vi "TestPython.vi"(8 "error in (no error)":errorcluster, 11 "Py Session":refnum<k35>) -> (0 "error out":errorcluster, 3 "Py Session out":refnum<k35>)   [LabVIEW 2022 SP3, in "DLP2.lvclass"]
uses:
  DLP2.lvclass
  DLP2.lvclass/DLP2.ctl
panel:
  out "return value":i32
  out "Cluster":cluster{"Error":bool, "Status":string}
  # "python PPP_app_CLI.py -t C30L -p DL_1 -ph 1 -m C30L -w 0.0898 -d 1.00 -o 1.15 -x 5 -n 735957 -f DB -l None -z True -c compensation_zone_list2.csv -b WBG_images\\DL_1_C30L.bmp -r True -s cwd\\Dithered_images -g cwd\\Saved_GS_images -ro True -dr \"SQL Server\" -se tt-local.digilens.com -db ToolTrack -u tooltrack-user -pa DigiLens_rEAd_passwrd"
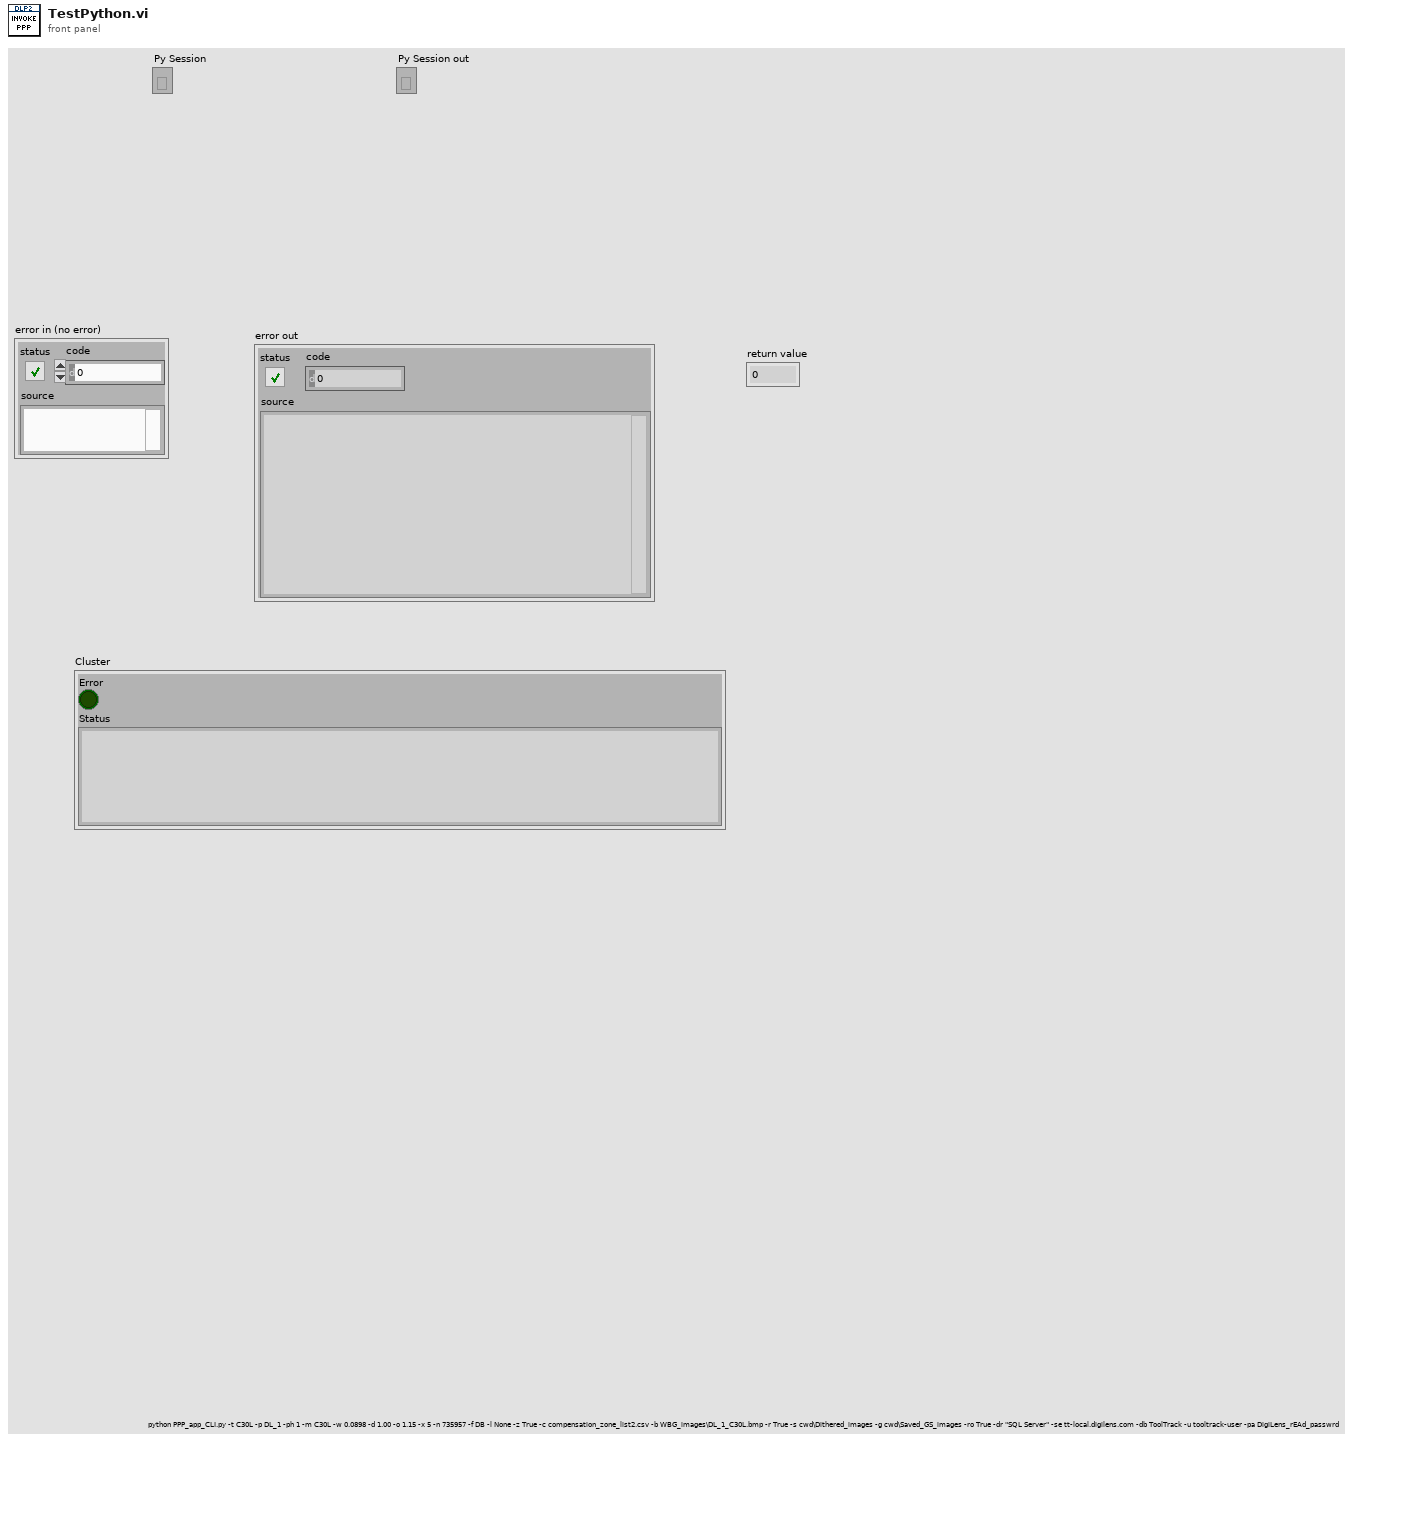
[diagram p1: front panel]
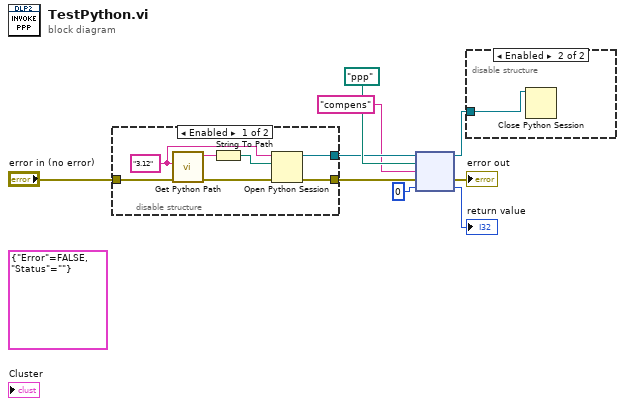
[diagram p0: block diagram]
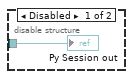
[diagram p2: hidden frame]
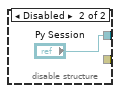
[diagram p3: hidden frame]
diagram:
  (unwired) cluster{"Error":bool, "Status":string} {"Error"=FALSE, "Status"=""}
  n1 = disable-structure shown="Enabled" {
    disable-tunnel: [w13 "Py Session"] -> w6
    disable-tunnel: [w12 _] -> w5
    disable-tunnel: "error in (no error)" -> [w10 _]
    frame Enabled {
      w14 = "3.12" ("Python Rev Key")
      n2 = call "Get Python Path.vi"("error in (no error)"=w10, "Python Rev Key"=w14) -> ("error out"=w11:errorcluster, "Python.exe path"=w16:string)  [unwired: 8 in]
      n3 = String To Path(string=w16) -> (path=w15:path)
      n4 = Open Python Session(python version=w14, python path=w15, 3:w11) -> (session out=w13:refnum<k35>, error out=w12:errorcluster)
    }
    frame Disabled {
    }
  }
  n5 = node(w6, path "ppp", "compens" ("function name"), w5, 0) -> (w9:refnum<k35>, →"error out":errorcluster, →"return value":i32)  [unwired: 2 out]
  n6 = disable-structure shown="Enabled" {
    disable-tunnel: w9 -> [w18 w19]
    frame Disabled {
      "Py Session out" <- w18
    }
    frame Enabled {
      n7 = Close Python Session(session in=w19) -> ()  [unwired: 1 in, 1 out]
    }
  }
